vi "Global - Configuration Options.vi"() -> ()   [LabVIEW 2018]
uses:
  controls/Trial Config Settings.ctl
  controls/Rig Config Settings.ctl
panel:
  in  "Slide":refnum<vi>
  in  "XY Graph":refnum<vi>
  in  "Hist Waveform Plot":refnum<vi>
  in  "Histogram Plot2":refnum<vi>
  in  "Histogram Plot1":refnum<vi>
  out "Event Log Save Path":path
  out "Rig Config Directory":path
  in  "Rig Config Settings":T1={"Rig Name"="", "Rig Room"="", "Base Directory"="", "Computer IP Address"="", "Globals Name"="", "Treatmill Str"="", "cRIO Test Data Dir"=path "", "ai"="", "ao"="", "dio"="", "A_calib_str_row1"="", "A_calib_str_row2"="", "A_calib_str_row3"="", "Zero_V_str"="", "step_V"="", "Sample Freq"="", "ai_threshold"="", "run_speed_thresh"="", "speed_time_length"="", "wall ball gain"="", "max wall pos"="", "max cor width"="", "Trial Config Directory"=path "C:/Whisker Tester/Trials", "Randomize Trials?"=FALSE}
  in  "Trial Config Settings":T2={"Trial Label"="", "Type"="", "Timeout (secs)"="", "Inter-Trial Interval (secs)"="", "Left Wall Enabled"=FALSE, "Right Wall Enabled"=FALSE, "Corridor Reset"=FALSE, "Default Wall Position"="", "Open Loop Change Positions"="", "Open Loop Values (mm)"="", "Corridor Width Change Positions"="", "Corridor Width Values (mm) "="", "Turn Change Positions"="0", "Turn Values (deg)"="", "Left Texture Change Positions"="", "Right Texture Change Positions"="", "Video Frames (fps)"="", "Water Enabled"=FALSE, "Water Trial Position"="", "Photostimulation"="", "Water Corridor Max"="", "Water Range"="", "Water Drop Size (ms)"="", "Water Reward Position"="", "Duration (cm)"="", "Left Texture Enabled"=FALSE, "Right Texture Enabled"=FALSE, "Ps Trial Period"="", "Ps Inter-Pulse-Interval (ms)"="", "Ps Peak Power"="", "Ps Pulse Duration (ms)"="", "ephys_clock freq (hz)"="", "frame_clock (hz)"="", "Plot Color (Lateral Dist vs Trial Fraction)"=0}
  out "Data Save Path":path
  in  "Error Log Duplicate Interval (ms)":u32=5000
  in  "Network Stream Polling Timeout (ms)":i32=500
  in  "Debugging":bool=TRUE
  in  "Error Log Max Size (bytes)":i64=100000
  in  "RT Error Log":path=path "c:/logs/log.txt"
  in  "Control Period (ticks)":u32=40000
  in  "Timeout Period (ticks)":u64=40000000
  in  "RT Stream Name":string="Command Stream from RT"
  in  "Monitoring Loop Rate (ms)":u32=200
  in  "Watchdog Pet Rate (ms)":u32=100
  in  "UI Stream Name":string="Command Stream from UI"
  in  "Network Stream Connect Timeout (ms)":i32=5000
  # "If you change any of these default configuration options, you must select Edit > Make Current Values Default before saving this VI."
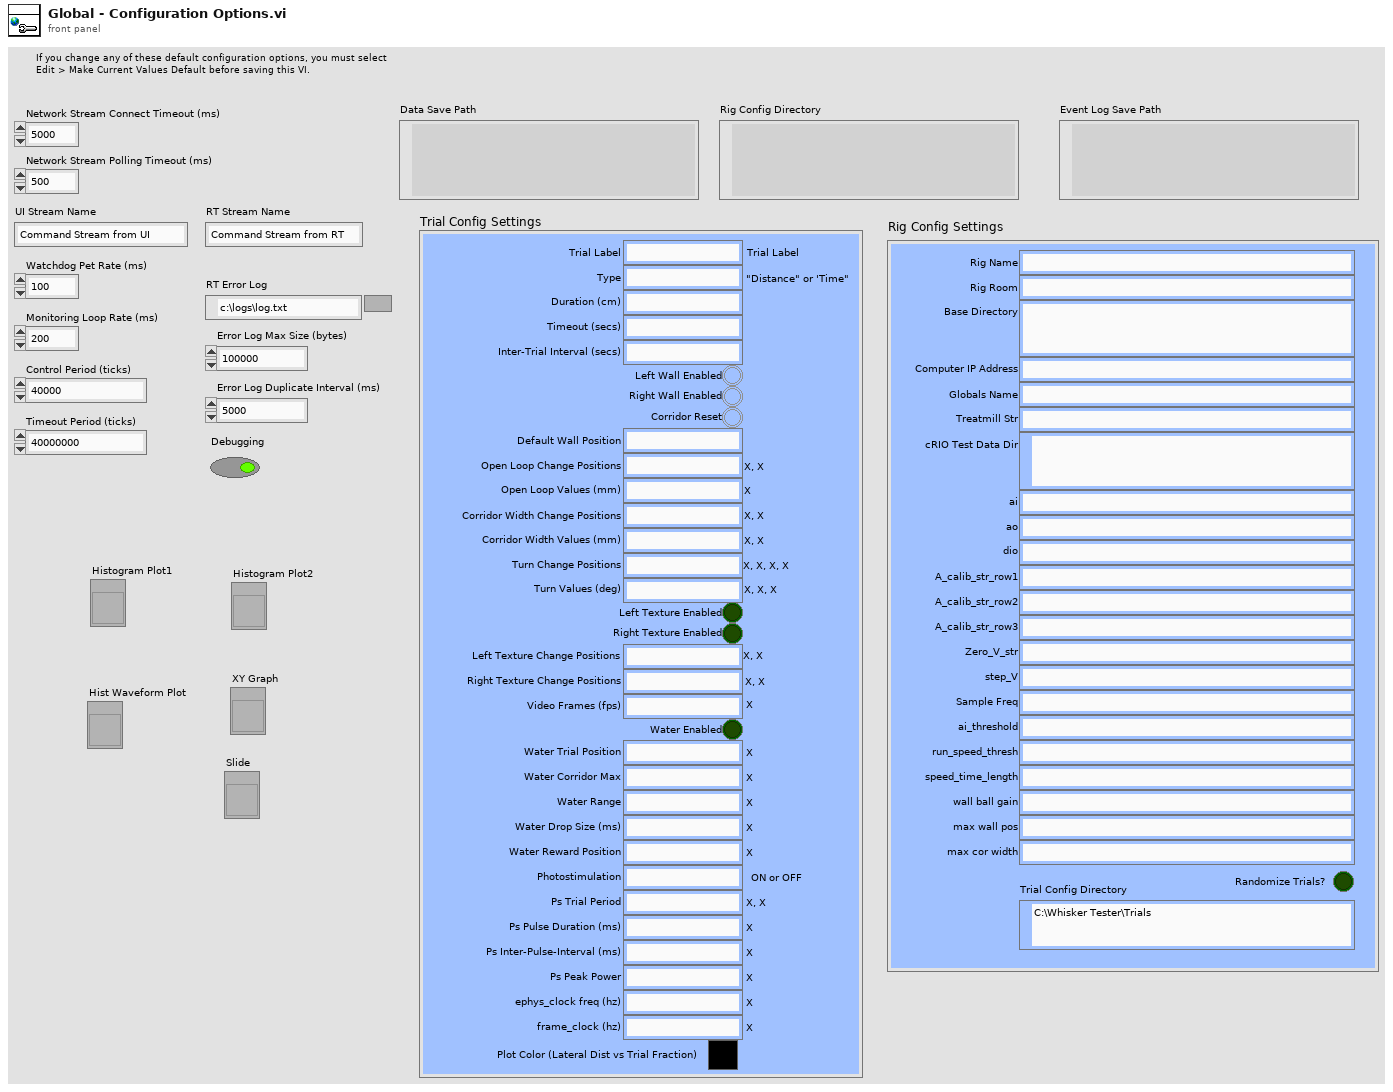
[diagram p1: front panel]
types:
  T1 = typedef "Rig Config Settings.ctl" = cluster{"Rig Name":string, "Rig Room":string, "Base Directory":string, "Computer IP Address":string, "Globals Name":string, "Treatmill Str":string, "cRIO Test Data Dir":path, "ai":string, "ao":string, "dio":string, "A_calib_str_row1":string, "A_calib_str_row2":string, "A_calib_str_row3":string, "Zero_V_str":string, "step_V":string, "Sample Freq":string, "ai_threshold":string, "run_speed_thresh":string, "speed_time_length":string, "wall ball gain":string, "max wall pos":string, "max cor width":string, "Trial Config Directory":path, "Randomize Trials?":bool}
  T2 = typedef "Trial Config Settings.ctl" = cluster{"Trial Label":string, "Type":string, "Timeout (secs)":string, "Inter-Trial Interval (secs)":string, "Left Wall Enabled":bool, "Right Wall Enabled":bool, "Corridor Reset":bool, "Default Wall Position":string, "Open Loop Change Positions":string, "Open Loop Values (mm)":string, "Corridor Width Change Positions":string, "Corridor Width Values (mm) ":string, "Turn Change Positions":string, "Turn Values (deg)":string, "Left Texture Change Positions":string, "Right Texture Change Positions":string, "Video Frames (fps)":string, "Water Enabled":bool, "Water Trial Position":string, "Photostimulation":string, "Water Corridor Max":string, "Water Range":string, "Water Drop Size (ms)":string, "Water Reward Position":string, "Duration (cm)":string, "Left Texture Enabled":bool, "Right Texture Enabled":bool, "Ps Trial Period":string, "Ps Inter-Pulse-Interval (ms)":string, "Ps Peak Power":string, "Ps Pulse Duration (ms)":string, "ephys_clock freq (hz)":string, "frame_clock (hz)":string, "Plot Color (Lateral Dist vs Trial Fraction)":u32}
diagram:
